vi "Initialize.vi"(8 "error in (no error)":errorcluster, 11 "Format Key Class in":refnum<class "Format Key Class.lvclass">) -> (0 "error out":errorcluster, 3 "Format Key Class out":refnum<class "Format Key Class.lvclass">)   [LabVIEW 2021, in "Library.lvlib" / "Format Key Class.lvclass"]
uses:
  Format Key Class.lvclass
  Format Key Class.lvclass/Format Key Class.ctl
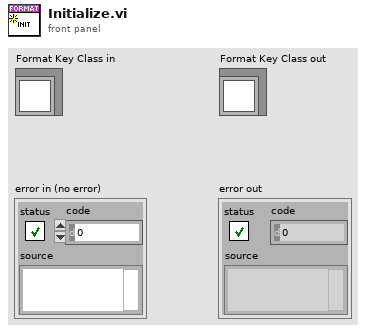
[diagram p1: front panel]
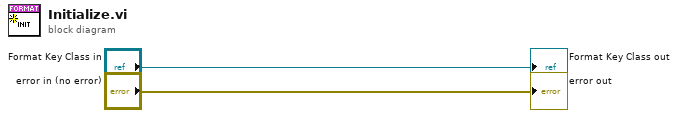
[diagram p0: block diagram]
diagram:
  "error out" <- "error in (no error)"
  "Format Key Class out" <- "Format Key Class in"
